vi "paticle处理.vi"(6 "ROI Descriptor":T2={"Global Rectangle"=[249, 829, 841, 1937], "Contours"=[{"ID"=enum."External", "Type"=12, "Coordinates"=[249, 829, 841, 1937, 0]}]} {"Contours"."Type" items=["No Selection", "Point", "Line", "Rectangle", "Oval", "Polygon", "Freehand Region", "Annulus", "Unused2", "Unused3", "Broken Line", "Freehand Line", "Rotated Rectangle"]}, 7 "Image Out 2":T1) -> (3 "Particle Measurements (Pixels)":dbl[][](array[numeric]) format="%.2f")   [LabVIEW 2014]
uses:
  <vilib>/vision/Image Controls.llb/IMAQ Image.ctl
  <vilib>/vision/NI_Vision_Development_Module.lvlib
panel:
  in  "File Path":path
  out "Image Out":T1(plugin-control)
  out "error out":errorcluster
  in  "error in":errorcluster
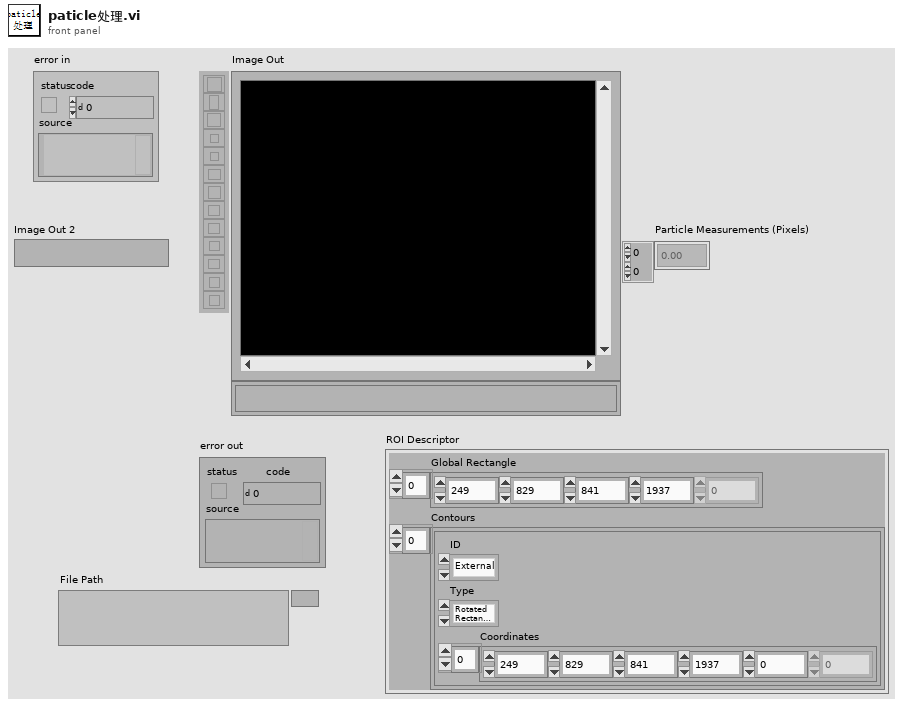
[diagram p1: front panel]
types:
  T1 = typedef "IMAQ Image.ctl" = refnum<image>
  T2 = cluster{"Global Rectangle":i32[], "Contours":cluster{"ID":enum32{"External", "Internal"}, "Type":u32, "Coordinates":i32[]}[]}
  T3 = cluster{"Measurement Parameter":i32, "Range Lower Value":dbl, "Range Upper Value":dbl, "Range":bool, "Measurement Type":bool}[]
  T4 = typedef "Image Type" = u32
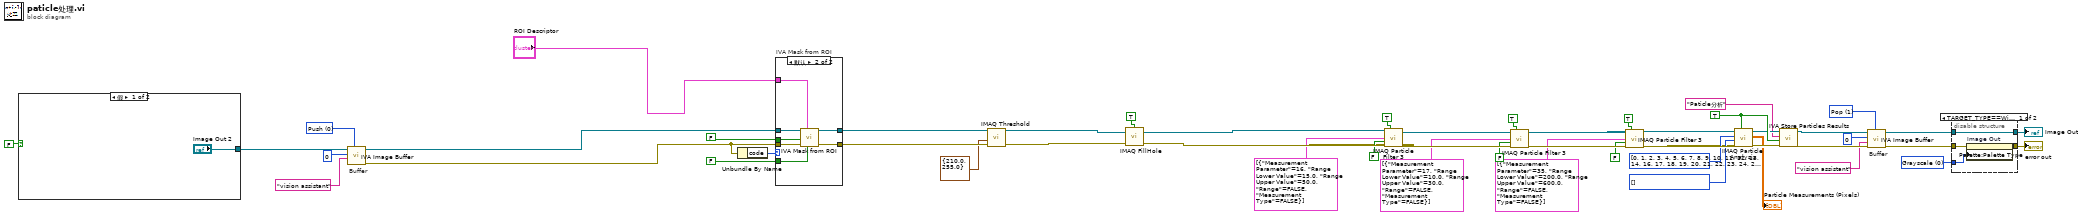
[diagram p0: block diagram]
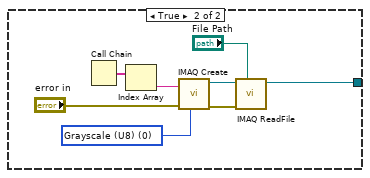
[diagram p2: hidden frame]
diagram:
  w3 = u32 0 items=["Grayscale", "Binary", "Gradient", "Rainbow", "Temperature", "User Defined"] ("Palette")
  w9 = u16 1 items=["Push", "Pop", "Reset"] ("Function")
  w18 = i32[] [] items=["Center of Mass X", "Center of Mass Y", "First Pixel X", "First Pixel Y", "Bounding Rect Left", "Bounding Rect Top", "Bounding Rect Right", "Bounding Rect Bottom", "Max Feret Diameter Start X", "Max Feret Diameter Start Y", "Max Feret Diameter End X", "Max Feret Diameter End Y", "Max Horiz. Segment Length Left", "Max Horiz. Segment Length Right", "Max Horiz. Segment Length Row", "-", "Bounding Rect Width", "Bounding Rect Height", "Bounding Rect Diagonal", "Perimeter", "Convex Hull Perimeter", "Holes' Perimeter", "Max Feret Diameter", "Equivalent Ellipse Major Axis", "Equivalent Ellipse Minor Axis", "Equivalent Ellipse Minor Axis (Feret)", "Equivalent Rect Long Side", "Equivalent Rect Short Side", "Equivalent Rect Diagonal", "Equivalent Rect Short Side (Feret)", "Average Horiz. Segment Length", "Average Vert. Segment Length", "Hydraulic Radius", "Waddel Disk Diameter", "-", "Area", "Holes' Area", "Particle & Holes' Area", "Convex Hull Area", "Image Area", "-", "Number of Holes", "Number of Horiz. Segments", "Number of Vert. Segments", "-", "Orientation", "Max Feret Diameter Orientation", "-", "% Area/Image Area", "% Area/(Particle & Holes' Area)", "Ratio of Equivalent Ellipse Axes", "Ratio of Equivalent Rect Sides", "-", "Elongation Factor", "Compactness Factor", "Heywood Circularity Factor", "Type Factor", "-", "Sum X", "Sum Y", "Sum XX", "Sum XY", "Sum YY", "Sum XXX", "Sum XXY", "Sum XYY", "Sum YYY", "-", "Moment of Inertia XX", "Moment of Inertia XY", "Moment of Inertia YY", "Moment of Inertia XXX", "Moment of Inertia XXY", "Moment of Inertia XYY", "Moment of Inertia YYY", "Norm. Moment of Inertia XX", "Norm. Moment of Inertia XY", "Norm. Moment of Inertia YY", "Norm. Moment of Inertia XXX", "Norm. Moment of Inertia XXY", "Norm. Moment of Inertia XYY", "Norm. Moment of Inertia YYY", "Hu Moment 1", "Hu Moment 2", "Hu Moment 3", "Hu Moment 4", "Hu Moment 5", "Hu Moment 6", "Hu Moment 7"] ("Real-World Measurements")
  w19 = i32[] [0, 1, 2, 3, 4, 5, 6, 7, 8, 9, 10, 11, 12, 13, 14, 16, 17, 18, 19, 20, 21, 22, 23, 24, 25, 26, 27, 28, 29, 30, 31, 32, 33, 35, 36, 37, 38, 39, 41, 42, 43, 45, 46, 48, 49, 50, 51, 53, 54, 55, 56, 58, 59, 60, 61, 62, 63, 64, 65, 66, 68, 69, 70, 71, 72, 73, 74, 75, 76, 77, 78, 79, 80, 81, 82, 83, 84, 85, 86, 87, 88] items=["Center of Mass X", "Center of Mass Y", "First Pixel X", "First Pixel Y", "Bounding Rect Left", "Bounding Rect Top", "Bounding Rect Right", "Bounding Rect Bottom", "Max Feret Diameter Start X", "Max Feret Diameter Start Y", "Max Feret Diameter End X", "Max Feret Diameter End Y", "Max Horiz. Segment Length Left", "Max Horiz. Segment Length Right", "Max Horiz. Segment Length Row", "-", "Bounding Rect Width", "Bounding Rect Height", "Bounding Rect Diagonal", "Perimeter", "Convex Hull Perimeter", "Holes' Perimeter", "Max Feret Diameter", "Equivalent Ellipse Major Axis", "Equivalent Ellipse Minor Axis", "Equivalent Ellipse Minor Axis (Feret)", "Equivalent Rect Long Side", "Equivalent Rect Short Side", "Equivalent Rect Diagonal", "Equivalent Rect Short Side (Feret)", "Average Horiz. Segment Length", "Average Vert. Segment Length", "Hydraulic Radius", "Waddel Disk Diameter", "-", "Area", "Holes' Area", "Particle & Holes' Area", "Convex Hull Area", "Image Area", "-", "Number of Holes", "Number of Horiz. Segments", "Number of Vert. Segments", "-", "Orientation", "Max Feret Diameter Orientation", "-", "% Area/Image Area", "% Area/(Particle & Holes' Area)", "Ratio of Equivalent Ellipse Axes", "Ratio of Equivalent Rect Sides", "-", "Elongation Factor", "Compactness Factor", "Heywood Circularity Factor", "Type Factor", "-", "Sum X", "Sum Y", "Sum XX", "Sum XY", "Sum YY", "Sum XXX", "Sum XXY", "Sum XYY", "Sum YYY", "-", "Moment of Inertia XX", "Moment of Inertia XY", "Moment of Inertia YY", "Moment of Inertia XXX", "Moment of Inertia XXY", "Moment of Inertia XYY", "Moment of Inertia YYY", "Norm. Moment of Inertia XX", "Norm. Moment of Inertia XY", "Norm. Moment of Inertia YY", "Norm. Moment of Inertia XXX", "Norm. Moment of Inertia XXY", "Norm. Moment of Inertia XYY", "Norm. Moment of Inertia YYY", "Hu Moment 1", "Hu Moment 2", "Hu Moment 3", "Hu Moment 4", "Hu Moment 5", "Hu Moment 6", "Hu Moment 7"] ("Pixel Measurements")
  w16 = TRUE ("Connectivity 4/8 (8)")
  w49 = u16 0 items=["Push", "Pop", "Reset"] ("Function")
  # "Buffer"
  # "Buffer"
  n1 = case shown="假" FALSE ("布尔") {
    tunnel: ["Image Out 2" w54] -> w51
    frame False {
    }
    frame True {
      w55 = T4 0 items=["Grayscale (U8)", "Grayscale (I16)", "Grayscale (SGL)", "Complex (CSG)", "RGB (U32)", "HSL (U32)", "RGB (U64)", "Grayscale (U16)"] ("Image Type")
      n2 = Call Chain() -> (call chain=w57:string[])
      n3 = Index Array(array=w57) -> (element=w56:string)  [unwired: 1 in]
      n4 = call "IMAQ Create"("Image Name"=w56, "Image Type"=w55, "error in (no error)"="error in") -> ("New Image"=w60:T1, "error out"=w59:errorcluster)  [unwired: 1 in, 1 out]
      n5 = call "IMAQ ReadFile"("File Path"="File Path", "error in (no error)"=w59, "Image"=w60) -> ("Image Out"=w54:T1)  [unwired: 2 in, 6 out]
    }
  }
  n6 = call <vilib>:"IVA Image Buffer.vi"("Function"=w49, "Prefix"="vision assistant", "Buffer #"=0, "Image In"=w51) -> ("error out"=w50:errorcluster, "Image Out"=w44:T1)  [unwired: 1 in, 5 out]
  n7 = Unbundle By Name(w50) -> ("code"=w41:i32)
  n8 = case "IVA Mask from ROI" shown="默认" w41 {
    tunnel: "ROI Descriptor" -> [_ w68]
    tunnel: FALSE ("Shrink") -> [_ w67]
    tunnel: w44 -> [w61 w66]
    tunnel: w50 -> [_ w65]
    tunnel: [_ w64] -> w43
    tunnel: [w61 w63] -> w39
    tunnel: FALSE ("Out / In") -> [_ w62]
    frame -1074396199, -1074396198 {
      # "Discard\nCoordinate\nSystem\nError"
    }
    frame Default {
      n9 = call <vilib>:"IVA Mask from ROI.vi"("Shrink"=w67, "ROI Descriptor"=w68, "error in (no error)"=w65, "Out / In"=w62, "Image Src"=w66) -> ("error out"=w64:errorcluster, "Image Out"=w63:T1)  [unwired: 5 out]
    }
  }
  n10 = call "IMAQ Threshold"("error in (no error)"=w43, "Range"=cluster{"Lower value":sgl, "Upper value":sgl} {"Lower value"=210.0, "Upper value"=255.0}, "Image Src"=w39) -> ("error out"=w38:errorcluster, "Image Dst Out"=w36:T1)  [unwired: 3 in, 4 out]
  n11 = call "IMAQ FillHole"("error in (no error)"=w38, "Image Src"=w36, "Connectivity 4/8 (8)"=TRUE) -> ("error out"=w35:errorcluster, "Image Dst Out"=w31:T1)  [unwired: 1 in, 2 out]
  n12 = call "IMAQ Particle Filter 3"("Image Src"=w31, "Connectivity 4/8 (8)"=TRUE, "Selection Values"=T3 [{"Measurement Parameter"=16, "Range Lower Value"=15.0, "Range Upper Value"=50.0, "Range"=FALSE, "Measurement Type"=FALSE}], "Keep/Remove Particles (F)"=FALSE ("Keep/Remove Particles"), "error in (no error)"=w35) -> ("Image Dst Out"=w26:T1, "error out"=w32:errorcluster)  [unwired: 4 in, 5 out]
  n13 = call "IMAQ Particle Filter 3"("Image Src"=w26, "Connectivity 4/8 (8)"=TRUE, "Selection Values"=T3 [{"Measurement Parameter"=17, "Range Lower Value"=10.0, "Range Upper Value"=30.0, "Range"=FALSE, "Measurement Type"=FALSE}], "Keep/Remove Particles (F)"=FALSE ("Keep/Remove Particles"), "error in (no error)"=w32) -> ("Image Dst Out"=w21:T1, "error out"=w27:errorcluster)  [unwired: 4 in, 5 out]
  n14 = call "IMAQ Particle Filter 3"("Image Src"=w21, "Connectivity 4/8 (8)"=TRUE, "Selection Values"=T3 [{"Measurement Parameter"=35, "Range Lower Value"=200.0, "Range Upper Value"=600.0, "Range"=FALSE, "Measurement Type"=FALSE}], "Keep/Remove Particles (F)"=FALSE ("Keep/Remove Particles"), "error in (no error)"=w27) -> ("Image Dst Out"=w17:T1, "error out"=w22:errorcluster)  [unwired: 4 in, 5 out]
  n15 = call "IMAQ Particle Analysis"("Connectivity 4/8 (8)"=w16, "error in (no error)"=w22, "Real-World Measurements"=w18, "Pixel Measurements"=w19, "Image"=w17) -> ("error out"=w13:errorcluster, "Particle Measurements (Pixels)"=→"Particle Measurements (Pixels)":dbl[][], "Image Out (duplicate)"=w15:T1)  [unwired: 4 out]
  n16 = call <vilib>:"IVA Store Particles Results.vi"("error in (no error)"=w13, "Connectivity 4/8 (8)"=w16, "Step Name"="Paticle分析", "Image in"=w15) -> ("error out"=w12:errorcluster, "Image dup"=w11:T1)  [unwired: 6 out]
  n17 = call <vilib>:"IVA Image Buffer.vi"("Function"=w9, "error in (no error)"=w12, "Prefix"="vision assistant", "Buffer #"=0, "Image In"=w11) -> ("error out"=w10:errorcluster, "Image Out"=w5:T1)  [unwired: 5 out]
  n18 = disable-structure "条件禁用结构" shown="TARGET_TYPE==Windows" {
    disable-tunnel: w10 -> [w72 w73]
    disable-tunnel: [w71 w73] -> w6
    disable-tunnel: w5 -> [w70 w74]
    disable-tunnel: [w70 w74] -> w4
    disable-tunnel: w3 -> [w69 _]
    frame condition #0 (active) {
      n19 = property on="Image Out" class="ImageControl"(error in=w72, "Palette:Palette Type"=w69) -> (error out=w71:errorcluster)  [unwired: 1 in, 1 out]
    }
    frame condition #1 {
    }
  }
  "error out" <- w6
  "Image Out" <- w4
